vi "ief_control_move_axis.vi"(3 "error in (no error)":errorcluster, 4 "Axis Number":u16=1 min=1 max=16, 5 "Tagprefix in":refnum<k21>) -> (0 "error out (no error)":errorcluster, 1 "Position":sgl format="%.2f", 2 "Tagprefix out":refnum<k21>)   [LabVIEW 2015, in "IEF Werner.lvlib"]
doc: "The VI is a supplement to the manual positioning commands and keeps the specified axis running. It has to be sent at least once in a second. Otherwise the manual positioning of the axis will be stopped. Furthermore it returns the present position of the chosen axis.\n\nAxis Number Range:\n01, 10 hex\n1, 16 dec"
uses:
  IEF Werner.lvlib
panel:
  # "IEF Control Move Axis"
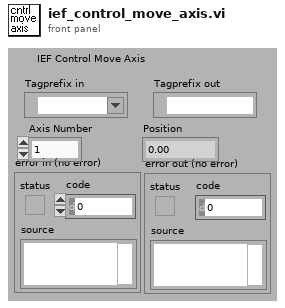
[diagram p1: front panel]
types:
  T1 = typedef "Semaphore RefNum" = refnum<k1>
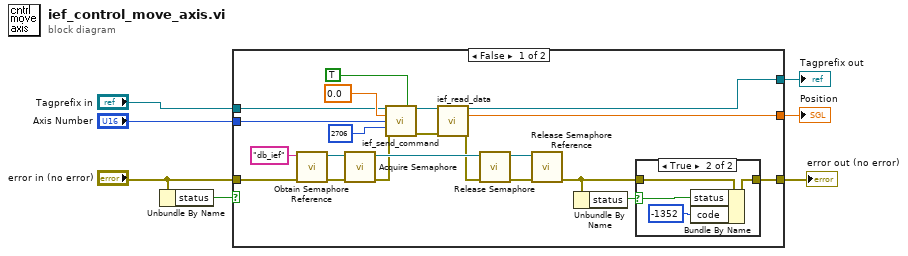
[diagram p0: block diagram]
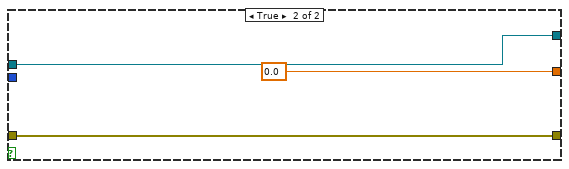
[diagram p3: hidden frame]
diagram:
  n1 = Unbundle By Name("error in (no error)") -> ("status"=w3:bool)
  n2 = case shown="False" w3 {
    tunnel: "error in (no error)" -> [w21 w36]
    tunnel: [w11 w36] -> w7
    tunnel: "Axis Number" -> [w18 _]
    tunnel: [w15 sgl 0.0 ("value real 32")] -> w5
    tunnel: "Tagprefix in" -> [w10 w35]
    tunnel: [w8 w35] -> w1
    frame False {
      n3 = call <vilib>:"Obtain Semaphore Reference.vi"("error in (no error)"=w21, "name (unnamed)"="db_ief") -> ("error out"=w26:errorcluster, "semaphore"=w27:T1)  [unwired: 3 in, 1 out]
      n4 = call <vilib>:"Acquire Semaphore.vi"("error in (no error)"=w26, "semaphore"=w27) -> ("error out"=w24:errorcluster, "semaphore out"=w25:T1)  [unwired: 3 in, 1 out]
      n5 = call "ief_send_command.vi"("Tagprefix in"=w10, "Command datum of type real"=TRUE, "Command datum"=sgl 0.0, "Command parameter"=w18, "Command code"=u16 2706, "error in (no error)"=w24) -> ("Tagprefix out"=w9:refnum<k21>, "error out (no error)"=w16:errorcluster)  [unwired: 4 in, 4 out]
      n6 = call "ief_read_data.vi"("Tagprefix in"=w9, "error in (no error)"=w16) -> ("Tagprefix out"=w8:refnum<k21>, "value real 32"=w15:sgl, "error out (no error)"=w14:errorcluster)  [unwired: 7 in, 4 out]
      n7 = call <vilib>:"Release Semaphore.vi"("error in (no error)"=w14, "semaphore"=w25) -> ("error out"=w23:errorcluster, "semaphore out"=w22:T1)  [unwired: 4 in]
      n8 = call <vilib>:"Release Semaphore Reference.vi"("error in (no error)"=w23, "semaphore"=w22) -> ("error out"=w12:errorcluster)  [unwired: 8 in, 1 out]
      n9 = Unbundle By Name(w12) -> ("status"=w13:bool)
      n10 = case shown="True" w13 {
        selector: w13 -> [_ w30]
        tunnel: [w29 w32] -> w11
        tunnel: w12 -> [w29 w33]
        frame False {
        }
        frame True {
          n11 = Bundle By Name(cluster=w33, "status"=w30, "code"=-1352) -> (w32:errorcluster)
        }
      }
    }
    frame True {
    }
  }
  "error out (no error)" <- w7
  "Position" <- w5
  "Tagprefix out" <- w1
